vi "NI PXIe-411x Change Name.vi"(8 "error in (no error)":errorcluster, 10 "New #":u16, 11 "Node Ptr":T1 format="%.0x") -> (0 "error out":errorcluster, 3 "Node Ptr out":T1 format="%.0x")   [LabVIEW 2023, in "NI PXIe-411x PS Custom Device.lvlib"]
uses:
  NI PXIe-411x PS Custom Device.lvlib
  <vilib>/NI VeriStand/Custom Device API/Custom Device Item Ref.ctl
  411x_Global.vi
  <vilib>/NI VeriStand/Custom Device API/Get Item Property (U16).vi
  <vilib>/NI VeriStand/Custom Device API/Custom Device API.lvlib
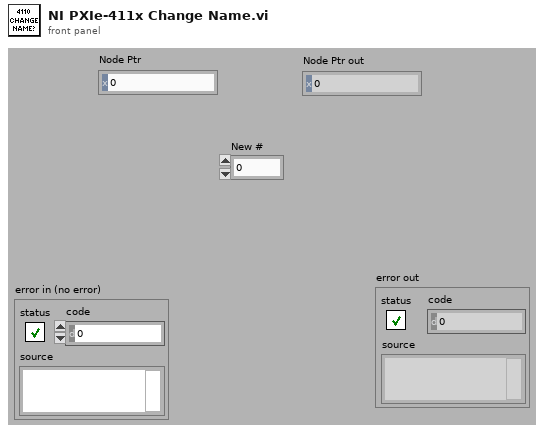
[diagram p1: front panel]
types:
  T1 = typedef "Custom Device API.lvlib/Custom Device Item Ref.ctl" = u64
  T2 = typedef "Custom Device API.lvlib/Custom Device Item Info.ctl" = cluster{"Name":string, "Is Channel":bool, "GUID":string, "Is Waveform":bool}
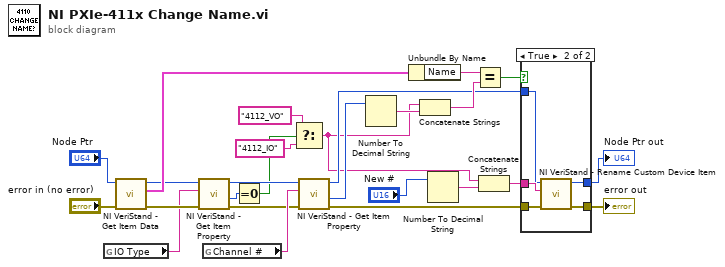
[diagram p0: block diagram]
diagram:
  n1 = global read "411x_Global.vi" "IO Type"() -> (w8:string)
  n2 = call <vilib>:"NI VeriStand - Get Item Data.vi"("error in (no error)"="error in (no error)", "Item Ref in"="Node Ptr") -> ("error out"=w10:errorcluster, "Item Info"=w25:T2, "Item Ref out"=w11:T1)  [unwired: 7 out]
  n3 = call-poly <vilib>:"NI VeriStand - Get Item Property.vi"("error in (no error)"=w10, "Property Name"=w8, "Item Ref in"=w11) -> ("error out"=w9:errorcluster, "Value"=w1:u16, "Item Ref out"=w7:T1)  [unwired: 5 in, 1 out]
  n4 = global read "411x_Global.vi" "Channel #"() -> (w12:string)
  n5 = Equal To 0?(x=w1) -> (x = 0?=w2:bool)
  n6 = Select(t="4112_VO" ("string"), s=w2, f="4112_IO" ("string")) -> (s? t:f=w4:string)
  n7 = call-poly <vilib>:"NI VeriStand - Get Item Property.vi"("error in (no error)"=w9, "Property Name"=w12, "Item Ref in"=w7) -> ("error out"=w19:errorcluster, "Value"=w23:u16, "Item Ref out"=w6:T1)  [unwired: 5 in, 1 out]
  n8 = Number To Decimal String(number=w23) -> (decimal integer string=w22:string)  [unwired: 1 in]
  n9 = Unbundle By Name(w25) -> ("Name"=w21:string)
  n10 = Concatenate Strings(w4, w22) -> (w20:string)
  n11 = Number To Decimal String(number="New #") -> (decimal integer string=w17:string)  [unwired: 1 in]
  n12 = Equal?(x=w21, y=w20) -> (x = y?=w13:bool)
  n13 = Concatenate Strings(w4, w17) -> (w16:string)
  n14 = case shown="True" w13 {
    tunnel: w19 -> [w28 w33]
    tunnel: w16 -> [_ w32]
    tunnel: w6 -> [w27 w31]
    tunnel: [w27 w30] -> w15
    tunnel: [w28 w29] -> w14
    frame False {
    }
    frame True {
      n15 = call <vilib>:"NI VeriStand - Rename Custom Device Item.vi"("error in (no error)"=w33, "New Name"=w32, "Item Ref in"=w31) -> ("error out"=w29:errorcluster, "Item Ref out"=w30:T1)  [unwired: 1 in, 6 out]
    }
  }
  "error out" <- w14
  "Node Ptr out" <- w15
